vi "Initialize.vi"(8 "error in (no error)":errorcluster, 9 "Data Cluster (for Headers)":variant, 10 "TableLogger Config":T1, 11 "object in":refnum<class "TableLogger_Actor.lvclass">) -> (0 "error out":errorcluster, 3 "object out":refnum<class "TableLogger_Actor.lvclass">)   [LabVIEW 2014, in "TableLogger_Actor.lvlib" / "TableLogger_Actor.lvclass"]
uses:
  TableLogger_Actor.lvclass
  TableLoggerConfig.ctl
  TableLoggerTypes.ctl
  TableLoggerBackupConfig.ctl
  TableLogger_Actor.lvclass/TableLogger_Actor.ctl
  TableLogger_Actor.lvlib
panel:
  # "Connector Pane"
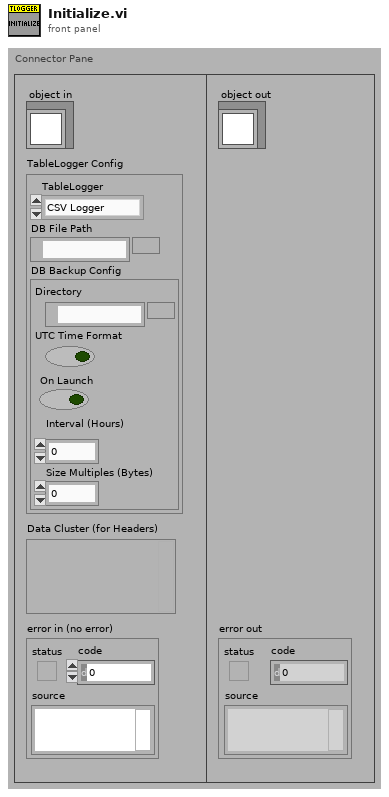
[diagram p1: front panel]
types:
  T1 = typedef "TableLogger_Actor.lvlib/TableLoggerConfig.ctl" = cluster{"TableLogger":T2, "DB File Path":path, "DB Backup Config":T3}
  T2 = typedef "TableLogger_Actor.lvlib/TableLoggerTypes.ctl" = enum16{"CSV Logger", "SQLite Logger"}
  T3 = typedef "TableLogger_Actor.lvlib/TableLoggerBackupConfig.ctl" = cluster{"Directory":path, "UTC Time Format":bool, "On Launch":bool, "Interval (Hours)":dbl, "Size Multiples (Bytes)":i32}
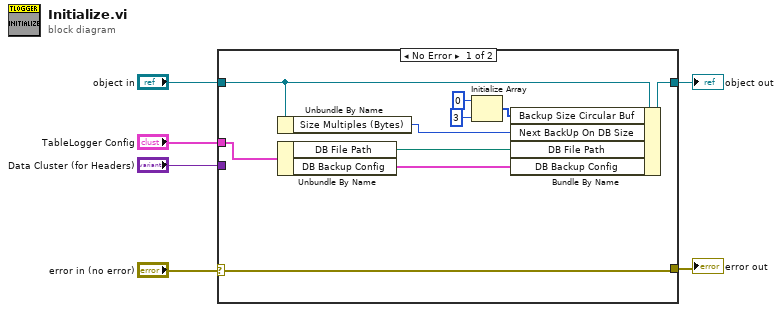
[diagram p0: block diagram]
diagram:
  n1 = case shown="No Error" "error in (no error)" {
    selector: "error in (no error)" -> [w16 w18]
    tunnel: [w16 w18] -> w6
    tunnel: [w15 w17] -> w5
    tunnel: "object in" -> [w11 w17]
    tunnel: "Data Cluster (for Headers)" -> [_ _]
    tunnel: "TableLogger Config" -> [w9 _]
    frame No Error {
      n2 = Unbundle By Name(w11) -> ("Size Multiples (Bytes)"=w10:i32)
      n3 = Unbundle By Name(w9) -> ("DB File Path"=w8:path, "DB Backup Config"=w7:T3)
      n4 = Initialize Array(0 ("element"), 3 ("dimension size")) -> (w14:i32[])
      n5 = Bundle By Name(cluster=w11, "Backup Size Circular Buf"=w14, "Next BackUp On DB Size"=w10, "DB File Path"=w8, "DB Backup Config"=w7) -> (w15:refnum<class "TableLogger_Actor.lvclass">)
    }
    frame Error {
    }
  }
  "error out" <- w6
  "object out" <- w5
